vi "Power Accuracy Stimulus Key Array.vi"(4 "Conversion":enum16{"Cluster - HTML", "HTML - Cluster"}(ring), 6 "Stimulus Key Array In":T2, 7 "Stimulus Cluster In":T1={"Power Start"=38, "Power Stop"=46, "Frequency Type"=enum."Band Edges", "Frequency Points"=[], "TX 1 Frequency (MHz)"={"Min"=0.0, "Max"=0.0}, "TX 2 Frequency (MHz)"={"Min"=0.0, "Max"=0.0}, "RX Frequency (MHz)"={"Min"=0.0, "Max"=0.0}, "Pad Model Number"="", "Pad Serial Number"="", "Pad Values"=[]}) -> (1 "Stimulus Cluster Out":T1={"Power Start"=38, "Power Stop"=46, "Frequency Type"=enum."Band Edges", "Frequency Points"=[], "TX 1 Frequency (MHz)"={"Min"=0.0, "Max"=0.0}, "TX 2 Frequency (MHz)"={"Min"=0.0, "Max"=0.0}, "RX Frequency (MHz)"={"Min"=0.0, "Max"=0.0}, "Pad Model Number"="", "Pad Serial Number"="", "Pad Values"=[]}, 2 "Stimulus HTML Out":string)   [LabVIEW 2011]
uses:
  ITK EXT/utils/keyedarr.llb/Keyed Array.ctl
  TypeDefs/Power Accuracy Stimulus Parameters.ctl
  ITK EXT/utils/strutil.llb/Case Matching.ctl
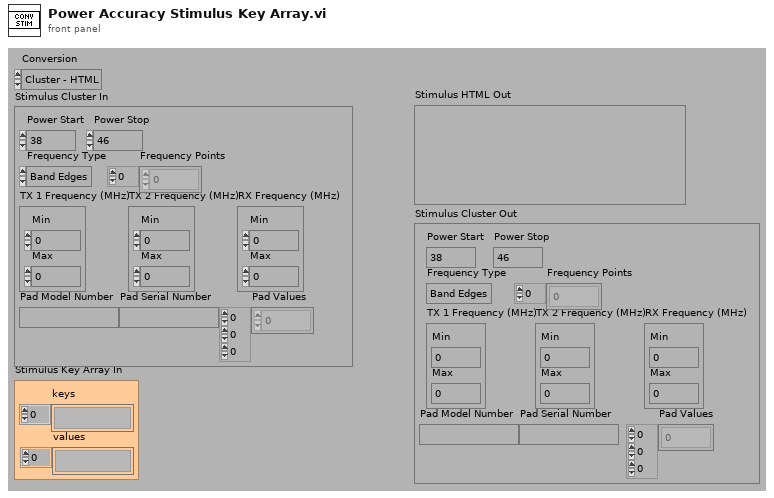
[diagram p1: front panel]
types:
  T1 = typedef "Power Accuracy Stimulus Parameters.ctl" = cluster{"Power Start":i32, "Power Stop":i32, "Frequency Type":enum16{"Band Edges", "Custom"}, "Frequency Points":dbl[], "TX 1 Frequency (MHz)":cluster{"Min":dbl, "Max":dbl}, "TX 2 Frequency (MHz)":cluster{"Min":dbl, "Max":dbl}, "RX Frequency (MHz)":cluster{"Min":dbl, "Max":dbl}, "Pad Model Number":string, "Pad Serial Number":string, "Pad Values":dbl[][][]}
  T2 = typedef "Keyed Array.ctl" = cluster{"keys":string[], "values":string[]}
  T3 = typedef "Case Matching.ctl" = enum16{"a != A", "a == A", "system"}
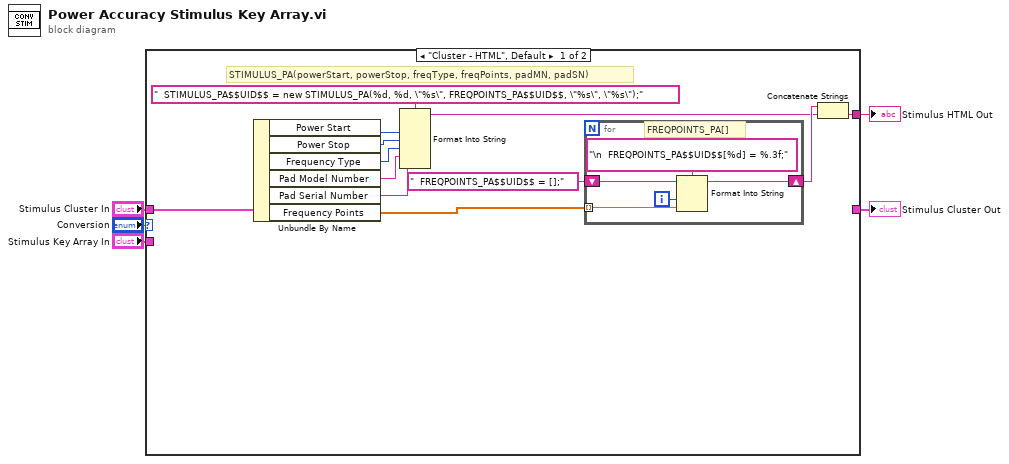
[diagram p0: block diagram]
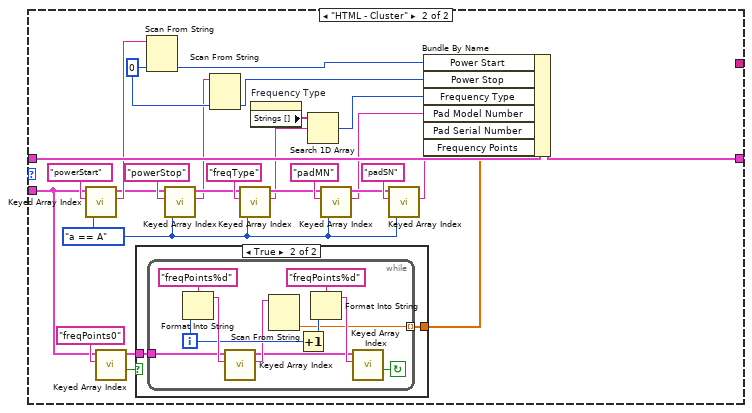
[diagram p2: hidden frame]
diagram:
  n1 = case shown="\"Cluster - HTML\", Default" "Conversion" {
    tunnel: "Stimulus Key Array In" -> [_ w24]
    tunnel: "Stimulus Cluster In" -> [w17 w48]
    tunnel: [w6 _] -> w3
    tunnel: [_ w47] -> w2
    frame "Cluster - HTML", Default {
      # "STIMULUS_PA(powerStart, powerStop, freqType, freqPoints, padMN, padSN)"
      n2 = Unbundle By Name(w17) -> ("Power Start"=w15:i32, "Power Stop"=w14:i32, "Frequency Type"=w13:enum16{"Band Edges", "Custom"}, "Pad Model Number"=w11:string, "Pad Serial Number"=w12:string, "Frequency Points"=w9:dbl[])
      n3 = Format Into String(format string="  STIMULUS_PA$$UID$$ = new STIMULUS_PA(%d, %d, \"%s\", FREQPOINTS_PA$$UID$$, \"%s\", \"%s\");", w15, w14, w13, w11, w12) -> (resulting string=w7:string)  [unwired: 2 in, 1 out]
      n4 = for {
        shift-right: [w20] -> w8
        shift-left: "  FREQPOINTS_PA$$UID$$ = [];" ("format string") -> [w21]
        tunnel: w9 -> [w18] mode=indexing
        i -> [w19]
        # "FREQPOINTS_PA[]"
        n5 = Format Into String(format string="\n  FREQPOINTS_PA$$UID$$[%d] = %.3f;", initial string=w21, w19, w18) -> (resulting string=w20:string)  [unwired: 1 in, 1 out]
      }
      n6 = Concatenate Strings(w8, w7) -> (w6:string)
    }
    frame "HTML - Cluster" {
      w36 = 0
      w33 = Case_Matching."a == A" ("case matching (sensitive)")
      n7 = call "Keyed Array Index.vi"("case matching (sensitive)"=w33, "key"="powerStart", "array in"=w24) -> ("value"=w39:string, "duplicate array"=w38:T2)  [unwired: 1 in, 2 out]
      n8 = call "Keyed Array Index.vi"("key"="freqPoints0", "array in"=w24) -> ("valid key"=w26:bool, "duplicate array"=w27:T2)  [unwired: 2 in, 2 out]
      n9 = case shown="True" w26 {
        tunnel: w27 -> [_ w51]
        tunnel: [_ w50] -> w23
        frame False {
        }
        frame True {
          n10 = while {
            tunnel: w51 -> [w55]
            tunnel: [w53] -> w50 mode=indexing
            i -> [w56]
            stop <- w59 continue-if-true
            n11 = Format Into String(format string="freqPoints%d", w56) -> (resulting string=w57:string)  [unwired: 2 in, 1 out]
            n12 = call "Keyed Array Index.vi"("key"=w57, "array in"=w55) -> ("value"=w54:string, "duplicate array"=w52:T2)  [unwired: 2 in, 2 out]
            n13 = Scan From String(input string=w54) -> (output 1=w53:dbl)  [unwired: 4 in, 3 out]
            n14 = Increment(x=w56) -> (x+1=w60:i32)
            n15 = Format Into String(format string="freqPoints%d", w60) -> (resulting string=w61:string)  [unwired: 2 in, 1 out]
            n16 = call "Keyed Array Index.vi"("key"=w61, "array in"=w52) -> ("valid key"=w59:bool)  [unwired: 2 in, 3 out]
          }
        }
      }
      n17 = Scan From String(input string=w39, default 1=w36) -> (output 1=w37:i32)  [unwired: 3 in, 3 out]
      n18 = call "Keyed Array Index.vi"("case matching (sensitive)"=w33, "key"="powerStop", "array in"=w38) -> ("value"=w35:string, "duplicate array"=w40:T2)  [unwired: 1 in, 2 out]
      n19 = Scan From String(input string=w35, default 1=w36) -> (output 1=w34:i32)  [unwired: 3 in, 3 out]
      n20 = call "Keyed Array Index.vi"("case matching (sensitive)"=w33, "key"="freqType", "array in"=w40) -> ("value"=w29:string, "duplicate array"=w42:T2)  [unwired: 1 in, 2 out]
      n21 = property on="Frequency Type" class="Enum (strict)"() -> ("Strings []"=w30:string[])  [unwired: 2 in, 2 out]
      n22 = Search 1D Array(1D array=w30, element=w29) -> (index of element=w28:i32)  [unwired: 1 out]
      n23 = call "Keyed Array Index.vi"("case matching (sensitive)"=w33, "key"="padMN", "array in"=w42) -> ("value"=w31:string, "duplicate array"=w45:T2)  [unwired: 1 in, 2 out]
      n24 = call "Keyed Array Index.vi"("case matching (sensitive)"=w33, "key"="padSN", "array in"=w45) -> ("value"=w32:string)  [unwired: 1 in, 3 out]
      n25 = Bundle By Name(cluster=w48, "Power Start"=w37, "Power Stop"=w34, "Frequency Type"=w28, "Pad Model Number"=w31, "Pad Serial Number"=w32, "Frequency Points"=w23) -> (w47:T1)
    }
  }
  "Stimulus HTML Out" <- w3
  "Stimulus Cluster Out" <- w2
